vi "Configure Time And Gain.vi"(0 "VISA Resource Name":refnum<visa-resource-name>, 1 "Filter Slope (0: No Filter)":u16(ring) items=["No Filter", "6 dB/oct", "12 dB/oct", "18 dB/oct", "24 dB/oct"], 2 "Time Constant (0:100 us)":u16(ring) items=["100 us", "300 us", "1 ms", "3 ms", "10 ms", "30 ms", "100 ms", "300 ms", "1 s", "3 s", "10 s", "30 s", "100 s", "300 s", "1 ks", "3 ks", "10 ks", "30 ks"], 3 "Settling Timeout (10.0)":dbl=10.0 format="%.2f", 5 "Sensitivity Mode (T: Automatically)":bool=TRUE, 7 "Sensitivity (0: 100 nVrms/-127dBm)":u16(ring) items=["100 nVrms/-127dBm", "300 nVrms/-117 dBm", "1 uVrms / -107 dBm", "3 uVrms / -97 dBm", "10 uVrms / -87dBm", "30 uVrms / -77 dBm", "100 uVrms / -67 dBm ", "300 uVrms / -57 dBm", "1mVrms / -47 dBm", "3 mVrms / -37 dBm", "10 mVrms / - 27 dBm", "30 mVrms / -7 dBm", "100 mVrms / -7 dBm", "300 mVrms / 3 dBm", "1 Vrms / 13 dBm"], 9 "Wait for Settling (T: Yes)":bool=TRUE, 11 "Error In (no error)":errorcluster, 12 "Close Reserve Mode (T: Automatically)":bool=TRUE, 13 "Close Reserve (0: High Reserve)":u16(ring) items=["High Reserve", "Normal ", "Low Noise"]) -> (4 "VISA Resource Name Out":refnum<visa-resource-name>, 15 "Error Out":errorcluster)   [LabVIEW 2010, in "Stanford Research 844.lvlib"]
doc: "This VI configures gain and time constant."
uses:
  <instrlib>/Stanford Research 844/Stanford Research 844.lvlib
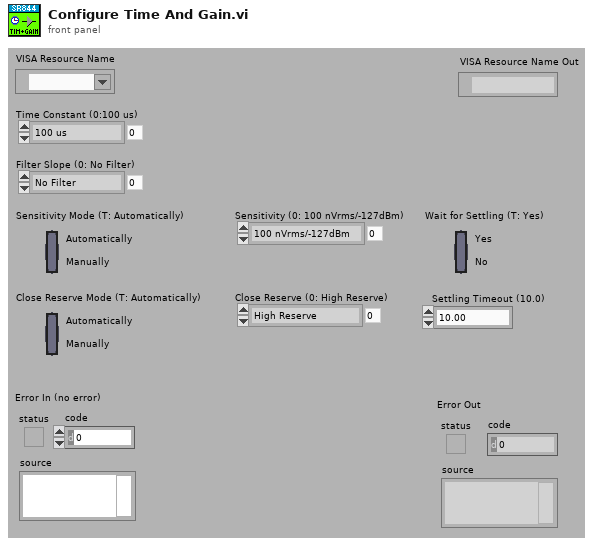
[diagram p1: front panel]
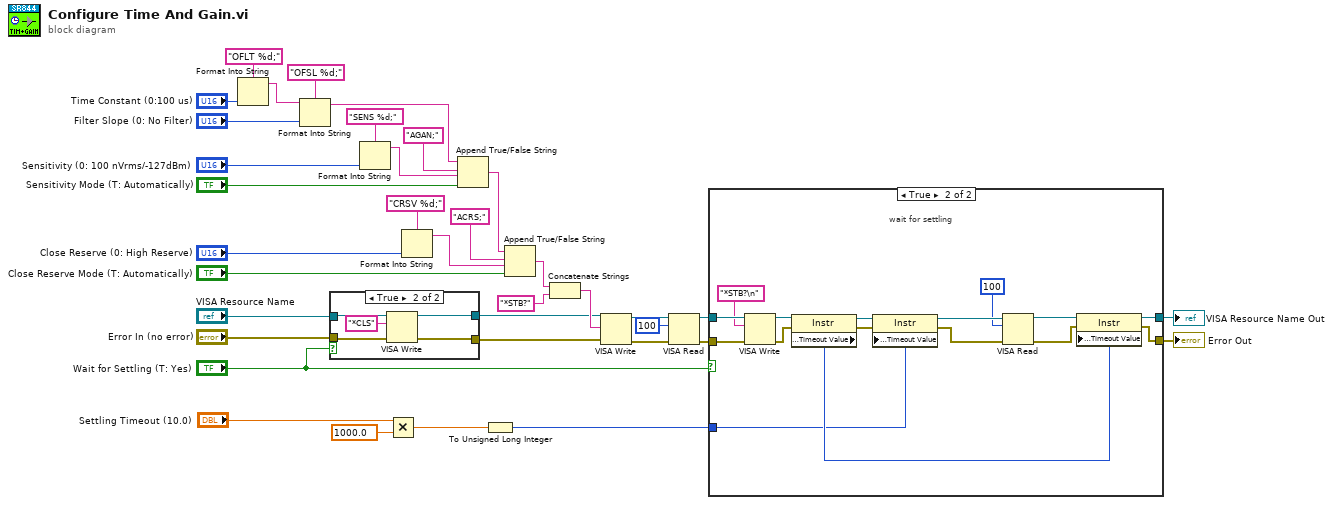
[diagram p0: block diagram]
diagram:
  n1 = Format Into String(format string="OFLT %d;", "Time Constant (0:100 us)") -> (resulting string=w22:string)  [unwired: 2 in, 1 out]
  n2 = Format Into String(format string="OFSL %d;", initial string=w22, "Filter Slope (0: No Filter)") -> (resulting string=w21:string)  [unwired: 1 in, 1 out]
  n3 = case shown="True" "Wait for Settling (T: Yes)" {
    tunnel: "VISA Resource Name" -> [w38 w43]
    tunnel: "Error In (no error)" -> [w37 w42]
    tunnel: [w37 w41] -> w14
    tunnel: [w38 w40] -> w13
    frame False {
    }
    frame True {
      n4 = VISA Write(VISA resource name=w43, write buffer="*CLS" ("write buffer (\"\")"), error in (no error)=w42) -> (VISA resource name out=w40:refnum<visa-resource-name>, error out=w41:errorcluster)  [unwired: 1 out]
    }
  }
  n5 = Format Into String(format string="SENS %d;", "Sensitivity (0: 100 nVrms/-127dBm)") -> (resulting string=w27:string)  [unwired: 2 in, 1 out]
  n6 = Multiply(x="Settling Timeout (10.0)", y=1000.0) -> (x*y=w4:dbl)
  n7 = Format Into String(format string="CRSV %d;" ("multi-line string"), "Close Reserve (0: High Reserve)") -> (resulting string=w23:string)  [unwired: 2 in, 1 out]
  n8 = Append True/False String(1:"Sensitivity Mode (T: Automatically)", 2:w27, 3:"AGAN;" ("write buffer (\"\")"), 4:w21) -> (0:w20:string)
  n9 = To Unsigned Long Integer(number=w4) -> (unsigned 32bit integer=w3:u32)
  n10 = Append True/False String(1:"Close Reserve Mode (T: Automatically)", 2:w23, 3:"ACRS;" ("write buffer (\"\")"), 4:w20) -> (0:w18:string)
  n11 = Concatenate Strings(w18, "*STB?" ("string")) -> (w17:string)
  n12 = VISA Write(VISA resource name=w13, write buffer=w17, error in (no error)=w14) -> (VISA resource name out=w7:refnum<visa-resource-name>, error out=w8:errorcluster)  [unwired: 1 out]
  n13 = VISA Read(VISA resource name=w7, byte count=u32 100 ("byte count (0)"), error in (no error)=w8) -> (VISA resource name out=w6:refnum<visa-resource-name>, error out=w5:errorcluster)  [unwired: 2 out]
  n14 = case shown="True" "Wait for Settling (T: Yes)" {
    tunnel: [w45 w56] -> w10
    tunnel: [w44 w46] -> w9
    tunnel: w6 -> [w45 w52]
    tunnel: w5 -> [w44 w51]
    tunnel: w3 -> [_ w50]
    frame False {
      # "don't wait for settling"
    }
    frame True {
      # "wait for settling"
      n15 = VISA Write(VISA resource name=w52, write buffer="*STB?\n" ("string"), error in (no error)=w51) -> (VISA resource name out=w54:refnum<visa-resource-name>, error out=w53:errorcluster)  [unwired: 1 out]
      n16 = property class="Instr"(reference=w54, error in=w53) -> (reference out=w61:refnum<visa-resource-name>, error out=w60:errorcluster, "General Settings:Timeout Value"=w55:u32)
      n17 = property class="Instr"(reference=w61, error in=w60, "General Settings:Timeout Value"=w50) -> (reference out=w59:refnum<visa-resource-name>, error out=w58:errorcluster)
      n18 = VISA Read(VISA resource name=w59, byte count=u32 100 ("byte count (0)"), error in (no error)=w58) -> (VISA resource name out=w57:refnum<visa-resource-name>, error out=w47:errorcluster)  [unwired: 2 out]
      n19 = property class="Instr"(reference=w57, error in=w47, "General Settings:Timeout Value"=w55) -> (reference out=w56:refnum<visa-resource-name>, error out=w46:errorcluster)
    }
  }
  "Error Out" <- w9
  "VISA Resource Name Out" <- w10
